vi "Status_Frame_Rate_Globals.vi"() -> ()   [LabVIEW 2020]
panel:
  in  "IMU_STATUS4(ms)":i16=200
  in  "IMU_STATUS11(ms)":i16=200
  in  "IMU_STATUS6(ms)":i16=200
  in  "IMU_STATUS9(ms)":i16=50
  in  "CANcoder_SensorData_Period(ms)":u8=200
  in  "STATUS2_Period(ms)":i32=200
  in  "STATUS1_Period(ms)":i32=200
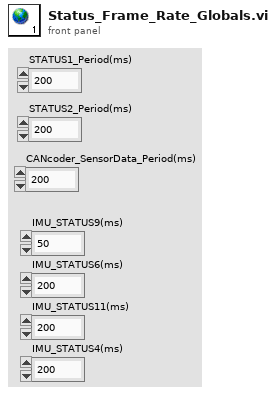
[diagram p1: front panel]
diagram:
